vi "DoubleAxisMoveAbsolute.vi"(4 "PositionY":dbl, 5 "PositionX":dbl, 6 "SpeedY":dbl, 7 "SpeedX":dbl, 9 "AxisName2":string, 11 "AxisName1":string) -> (1 "Y Absolute Position":string, 3 "X Absolute Positon":string)   [LabVIEW 2016]
uses:
  Examples/Motion/EnableMultiple.vi
  Examples/Motion/MoveAbsMultiple.vi
  Examples/Motion/WaitMultiple.vi
  Examples/Motion/DisableMultiple.vi
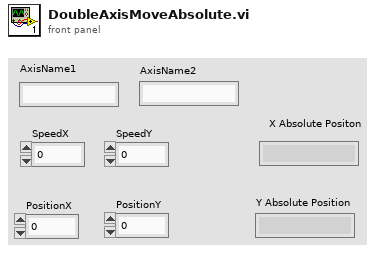
[diagram p1: front panel]
types:
  T1 = typedef "ControllerDiagPacket.ctl" = cluster{"Number of Diag Packets":i32, "Axes":T2[], "error":errorcluster}
  T2 = typedef "AxisDiagPacket.ctl" = cluster{"Axis Name":string, "Analog Input 0":dbl, "Analog Input 1":dbl, "Axis Fault (num)":i32, "Axis Fault (str)":string, "Axis Fault (bits)":cluster{"AmplifierFault":bool, "AmplifierTemperatureFault":bool, "CcwEndOfTravelLimitFault":bool, "CcwSoftwareLimitFault":bool, "CommunicationLostFault":bool, "CwEndOfTravelLimitFault":bool, "CwSoftwareLimitFault":bool, "EmergencyStopFault":bool, "EncoderFault":bool, "ExternalFault":bool, "FeedbackScalingFault":bool, "GantryMisalignFault ":bool, "HallSensorFault":bool, "InPositionTimeoutFault":bool, "MarkerSearchFault":bool, "MaxVelocityCommandFault":bool, "MissedInterruptFault":bool, "MotorTemperatureFault":bool, "None":bool, "OverCurrentFault":bool, "PositionErrorFault":bool, "PositionFeedbackFault":bool, "PowerSupplyFault":bool, "ProbeInputFault":bool, "SafeZoneFault":bool, "VelocityErrorFault":bool, "VelocityFeedbackFault":bool, "VoltageClampFault":bool}, "Axis Status (num)":i32, "Axis Status (str)":string, "Axis Status (bits)":cluster{"BacklashActive":bool, "CalibrationEnabled1D":bool, "CalibrationEnabled2D":bool, "CommandValid":bool, "DriveAbortPending":bool, "DrivePending":bool, "Enabling":bool, "GainMappingEnabled":bool, "GantryAligned":bool, "GantryRealigning":bool, "Homed":bool, "Homing":bool, "IFOVEnabled":bool, "JogGenerating":bool, "Jogging":bool, "JoystickControl":bool, "MasterSlaveControl":bool, "MotionBlocked":bool, "MotionClamped":bool, "MoveDone":bool, "None":bool, "NotVirtual":bool, "Profiling":bool, "Stability0":bool, "Stability1":bool, "TrajectoryFiltering":bool, "WaitDone":bool}, "Current Command":sgl, "Current Error":sgl, "Current Feedback":sgl, "Digital Inputs":i32, "Digital Outputs":i32, "Drive Status":i32, "Drive Status (str)":string, "Drive Status (bits)":cluster{"AccelerationPhase":bool, "AutofocusActive":bool, "BrakeOutput":bool, "CcwEndOfTravelLimitInput":bool, "CosineEncoderError":bool, "CurrentClamp":bool, "CwEndOfTravelLimitInput":bool, "DecelerationPhase":bool, "DualLoopActive":bool, "EmergencyStopInput":bool, "Enabled":bool, "EncoderClipping":bool, "GalvoCalibrationEnabled":bool, "GalvoPowerCorrection":bool, "HallAInput":bool, "HallBInput":bool, "HallCInput":bool, "HighResolutionMode":bool, "HomeLimitInput":bool, "InPosition":bool, "InPosition2":bool, "MarkerInput":bool, "MarkerLatch":bool, "MoveActive":bool, "NoMotorSupply":bool, "None":bool, "PowerLimiting":bool, "ProgrammingFlash":bool, "ProgrammingMXH":bool, "PSOHaltLatch":bool, "ServoControl":bool, "SineEncoderError":bool}, "Position Feedback Auxiliary":dbl, "Position Command":dbl, "Position Error":dbl, "Position Feedback":dbl, "Program Position Command":dbl, "Program Position Error":dbl, "Program Position Feedback":dbl, "Velocity Command":dbl, "Velocity Error":dbl, "Velocity Feedback":dbl}
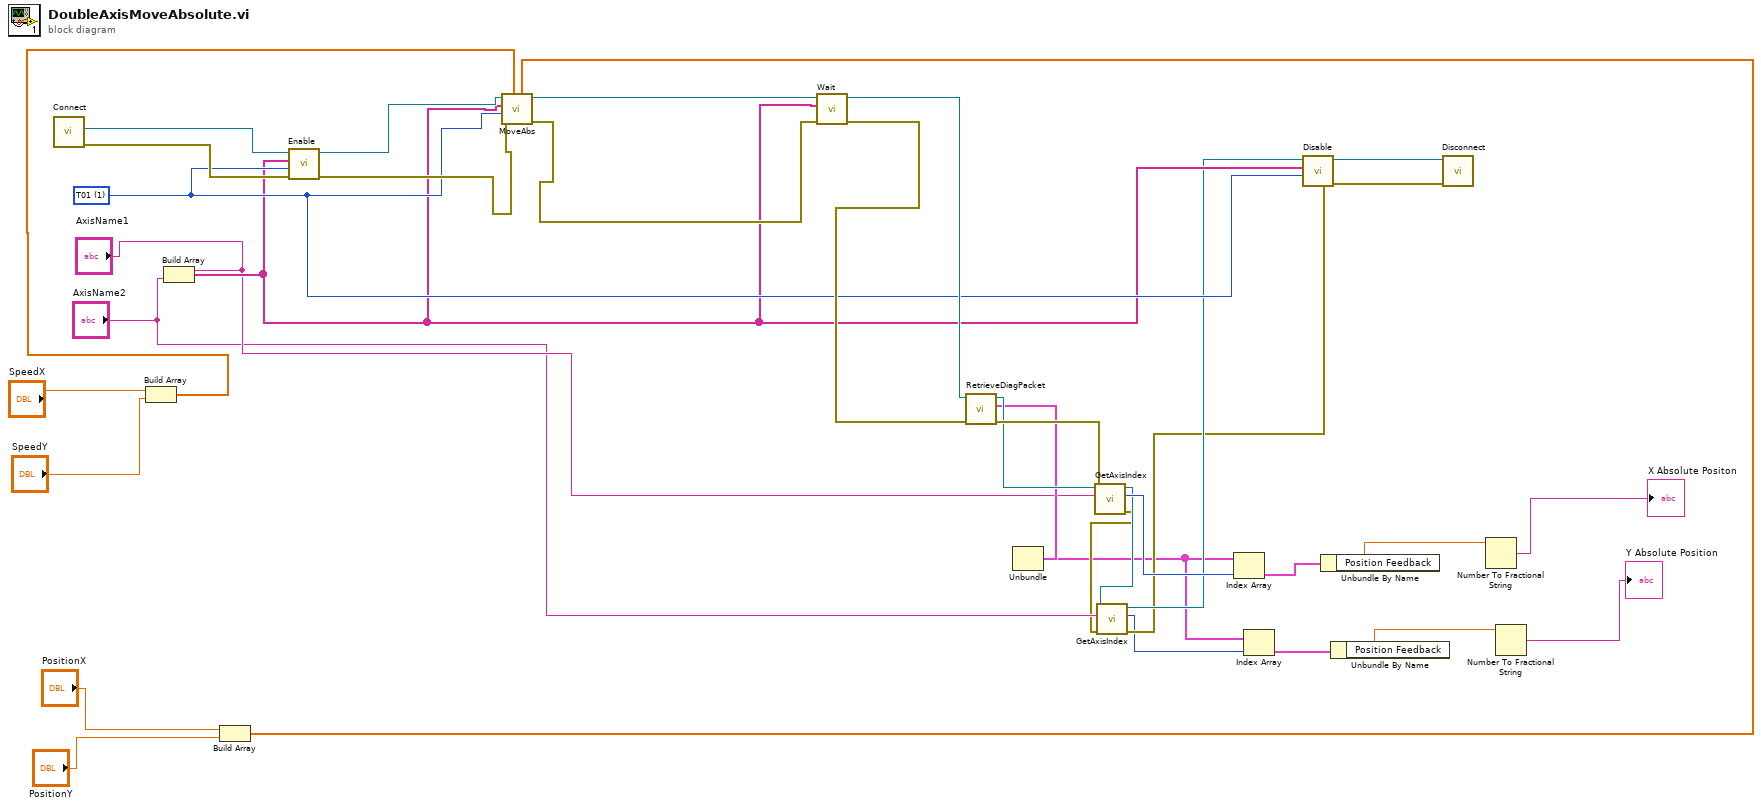
[diagram p0: block diagram]
diagram:
  w13 = 1 items=["TLibrary", "T01", "T02", "T03", "T04", "T05", "T06", "T07", "T08", "T09", "T10", "T11", "T12", "T13", "T14", "T15", "T16", "T17", "T18", "T19", "T20", "T21", "T22", "T23", "T24", "T25", "T26", "T27", "T28", "T29", "T30", "T31"] ("taskId")
  n1 = call "Connect.vi"() -> ("error out"=w35:errorcluster, "controller"=w36:refnum<k24>)  [unwired: 10 in]
  n2 = Build Array("SpeedX", "SpeedY") -> (w18:dbl[])
  n3 = Build Array("AxisName1", "AxisName2") -> (w12:string[])
  n4 = Build Array("PositionX", "PositionY") -> (w19:dbl[])
  n5 = call-poly "Enable.vi"("error in (no error)"=w35, "taskId"=w13, "axis names"=w12, "controller in"=w36) -> ("error out"=w14:errorcluster, "controller out"=w17:refnum<k24>)  [unwired: 6 in]
  n6 = call-poly "MoveAbs.vi"("positions"=w19, "speeds"=w18, "error in (no error)"=w14, "taskId"=w13, "axis names"=w12, "controller in"=w17) -> ("error out"=w15:errorcluster, "controller out"=w16:refnum<k24>)  [unwired: 4 in]
  n7 = call-poly "Wait.vi"("error in (no error)"=w15, "axis names"=w12, "controller in"=w16) -> ("error out"=w32:errorcluster, "controller out"=w30:refnum<k24>)  [unwired: 6 in, 1 out]
  n8 = call "RetrieveDiagPacket.vi"("error in (no error)"=w32, "Controller In"=w30) -> ("error out"=w31:errorcluster, "ControllerDiagPacket"=w28:T1, "Controller Out"=w29:refnum<k24>)  [unwired: 7 in]
  n9 = Unbundle(w28) -> ("Axes"=w5:T2[])  [unwired: 2 out]
  n10 = call "GetAxisIndex.vi"("error in (no error)"=w31, "axis name"="AxisName1", "controller in"=w29) -> ("error out"=w7:errorcluster, "axis index"=w27:i32, "controller out"=w9:refnum<k24>)  [unwired: 6 in]
  n11 = call "GetAxisIndex.vi"("error in (no error)"=w7, "axis name"="AxisName2", "controller in"=w9) -> ("error out"=w6:errorcluster, "axis index"=w4:i32, "controller out"=w8:refnum<k24>)  [unwired: 6 in]
  n12 = Index Array(array=w5, index=w27) -> (element=w26:T2)
  n13 = Index Array(array=w5, index=w4) -> (element=w2:T2)
  n14 = call-poly "Disable.vi"("error in (no error)"=w6, "taskId"=w13, "axis names"=w12, "controller in"=w8) -> ("error out"=w33:errorcluster, "controller out"=w34:refnum<k24>)  [unwired: 6 in]
  n15 = Unbundle By Name(w26) -> ("Position Feedback"=w25:dbl)
  n16 = Unbundle By Name(w2) -> ("Position Feedback"=w3:dbl)
  n17 = call "Disconnect.vi"("error in (no error)"=w33, "controller"=w34) -> ()  [unwired: 9 in, 1 out]
  n18 = Number To Fractional String(number=w25) -> (F-format string=→"X Absolute Positon":string)  [unwired: 3 in]
  n19 = Number To Fractional String(number=w3) -> (F-format string=→"Y Absolute Position":string)  [unwired: 3 in]
